vi "Poll Sample Transfer Control.vi"(8 "error in (no error)":errorcluster, 11 "cRIO-CO2 in":refnum<class "cRIO-CO2.lvclass">) -> (0 "error out":errorcluster, 3 "cRIO-CO2 out":refnum<class "cRIO-CO2.lvclass">)   [LabVIEW 2015, in "cRIO-Carbondioxide.lvlib" / "cRIO-CO2.lvlib" / "cRIO-CO2.lvclass"]
uses:
  cRIO-CO2.lvclass
  Controls/Sample Transfer Control Enumerator.ctl
  cRIO-CO2.lvclass/cRIO-CO2.ctl
  <vilib>/ActorFramework/Message Enqueuer/Message Enqueuer.lvclass/Message Enqueuer.ctl
  cRIO-CO2 Messages/Sample Transfer Reset to Idle Msg/Sample Transfer Reset to Idle Msg.lvclass/Sample Transfer Reset to Idle Msg.ctl
  cRIO-CO2 Messages/Initiate Sample Transfer Msg/Initiate Sample Transfer Msg.lvclass/Initiate Sample Transfer Msg.ctl
  <vilib>/ActorFramework/Message Enqueuer/Enqueue.vi
  <vilib>/ActorFramework/Message Priority Queue/Priority Enqueue.vi
  cRIO-CO2 Messages/Abort Sample Transfer Msg/Abort Sample Transfer Msg.lvclass
  cRIO-CO2 Messages/Sample Transfer Reset to Idle Msg/Sample Transfer Reset to Idle Msg.lvclass
  cRIO-CO2 Messages/Initiate Sample Transfer Msg/Initiate Sample Transfer Msg.lvclass
  cRIO-CO2 Messages/Sample Transfer Initiate Stash Msg/Sample Transfer Initiate Stash Msg.lvclass
panel:
  out "error IO":errorcluster
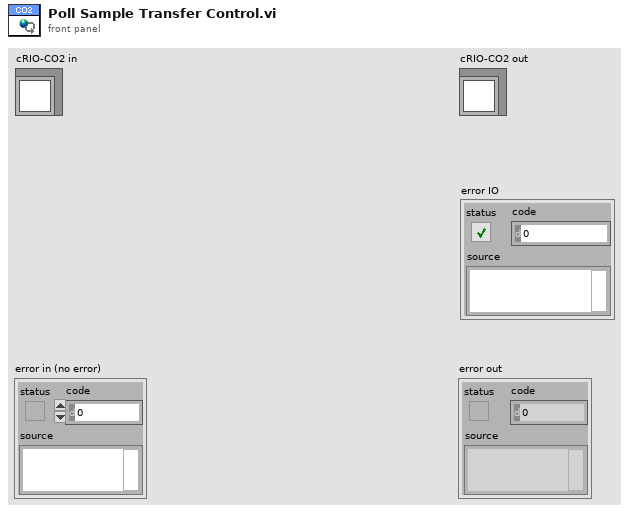
[diagram p1: front panel]
types:
  T1 = typedef "Sample Transfer Control Enumerator.ctl" = enum16{"Acknowledged", "Transfer", "Stash", "Abort", "Reset to Idle"}
  T2 = typedef "Sample Transfer Container Enumerator.ctl" = enum16{"None", "Sample 1", "Sample 2", "Sample 3", "Sample 4", "Sample 5", "Storage 01", "Storage 02", "Storage 03", "Storage 04", "Storage 05", "Storage 06", "Storage 07", "Storage 08", "Storage 09", "Storage 10", "Storage 11", "Storage 12", "Syringe", "Undefined"}
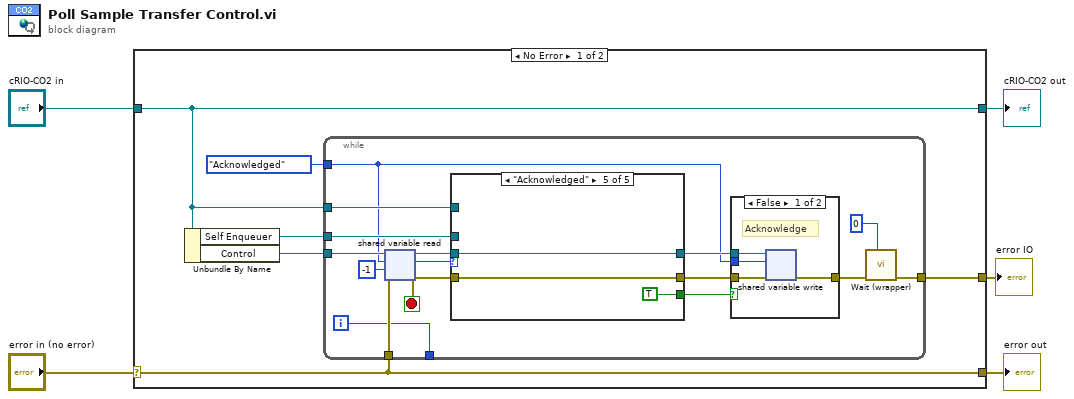
[diagram p0: block diagram]
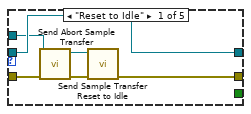
[diagram p3: hidden frame]
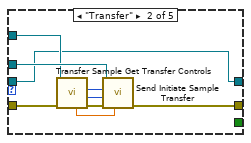
[diagram p4: hidden frame]
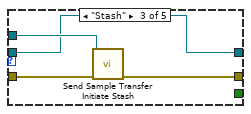
[diagram p5: hidden frame]
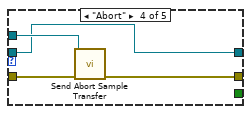
[diagram p6: hidden frame]
diagram:
  n1 = case shown="No Error" "error in (no error)" {
    selector: "error in (no error)" -> [w10 w60]
    tunnel: [w10 w60] -> w4
    tunnel: [w8 w59] -> w2
    tunnel: "cRIO-CO2 in" -> [w8 w59]
    tunnel: [w7 _] -> w1
    frame No Error {
      n2 = Unbundle By Name(w8) -> ("Self Enqueuer"=w9:refnum<class "Message Enqueuer.lvclass">, "Control"=w11:refnum<k21>)
      n3 = while {
        tunnel: w11 -> [w26]
        tunnel: w10 -> [w25]
        tunnel: Sample_Transfer_Control_Enumerator."Acknowledged" ("Sample Transfer Control") -> [w17]
        tunnel: [w15] -> w7
        tunnel: w9 -> [w21]
        tunnel: w8 -> [w19]
        tunnel: [w14] -> _
        i -> [w14]
        stop <- w23 stop-if-true
        n4 = shared-variable-read(w26, w25, w17, -1 ("timeout ms")) -> (w22:refnum<k21>, w23:errorcluster, w24:T1)  [unwired: 2 out]
        n5 = case shown="\"Acknowledged\"" w24 {
          tunnel: w23 -> [w38 w45 w51 w55 w58]
          tunnel: [w34 w47 w50 w54 w58] -> w18
          tunnel: w22 -> [w37 w39 w48 w52 w57]
          tunnel: [w37 w39 w48 w52 w57] -> w20
          tunnel: w21 -> [w36 w46 w49 w53 _]
          tunnel: w19 -> [_ w43 _ _ _]
          tunnel: [_ _ _ _ TRUE] -> w13
          frame "Reset to Idle" {
            n6 = call "Send Abort Sample Transfer.vi"("error in (no error)"=w38, "Message Enqueuer"=w36) -> ("error out"=w35:errorcluster, "Message Enqueuer out"=w33:refnum<class "Message Enqueuer.lvclass">)  [unwired: 8 in]
            n7 = call "Send Sample Transfer Reset to Idle.vi"("error in (no error)"=w35, "Message Enqueuer"=w33) -> ("error out"=w34:errorcluster)  [unwired: 8 in, 1 out]
          }
          frame "Transfer" {
            n8 = call "Transfer Sample Get Transfer Controls.vi"("error in (no error)"=w45, "cRIO-CO2 in"=w43) -> ("error out"=w44:errorcluster, "Target Container"=w41:T2, "Source Container"=w42:T2, "Transfer mBar"=w40:dbl)  [unwired: 5 in, 1 out]
            n9 = call "Send Initiate Sample Transfer.vi"("Transfer mBar"=w40, "error in (no error)"=w44, "Target Container"=w41, "Source Container"=w42, "Message Enqueuer"=w46) -> ("error out"=w47:errorcluster)  [unwired: 5 in, 1 out]
          }
          frame "Stash" {
            n10 = call "Send Sample Transfer Initiate Stash.vi"("error in (no error)"=w51, "Message Enqueuer"=w49) -> ("error out"=w50:errorcluster)  [unwired: 8 in, 1 out]
          }
          frame "Abort" {
            n11 = call "Send Abort Sample Transfer.vi"("error in (no error)"=w55, "Message Enqueuer"=w53) -> ("error out"=w54:errorcluster)  [unwired: 8 in, 1 out]
          }
          frame "Acknowledged" {
          }
        }
        n12 = case shown="False" w13 {
          tunnel: w20 -> [w31 _]
          tunnel: w18 -> [w30 w32]
          tunnel: w17 -> [w29 _]
          tunnel: [w28 w32] -> w16
          frame False {
            # "Acknowledge"
            n13 = shared-variable-write(w31, w30, w29) -> (w28:errorcluster)  [unwired: 1 out]
          }
          frame True {
          }
        }
        n14 = call "Wait (wrapper).vi"("milliseconds to wait (200)"=u32 0, "error in (no error)"=w16) -> ("error out"=w15:errorcluster)  [unwired: 9 in]
      }
    }
    frame Error {
    }
  }
  "error out" <- w4
  "cRIO-CO2 out" <- w2
  "error IO" <- w1
